vi "Get.vi"(8 "error in (no error)":errorcluster, 10 "uService ID":string, 11 "Distr uS Map ref in":refnum<data-value>) -> (0 "error out":errorcluster, 1 "uService found?":bool=TRUE, 2 "Guardians":string[](array[string]), 3 "Distr uS Map ref out":refnum<data-value>)   [LabVIEW 2026, in "TALOS.lvlib" / "Classes.lvlib" / "Distributed uService Map.lvclass"]
uses:
  Distributed uService Map.lvclass
  Distributed uService Map.lvclass/Distributed uService Map.ctl
  Ancestor/Ancestor/Ancestor.lvclass/Ancestor.ctl
  FGV/Error Memory/Get Error Description.vi
  Support VIs/Get PC name.vi
  Ancestor/Ancestor/Read ID.vi
  Support VIs/Get Class Name.vi
  <vilib>/Utility/error.llb/Clear Errors.vi
  FGV/Error Memory/Error Memory Core.vi
  <vilib>/AdvancedString/Delimited String to 1D String Array.vi
  <vilib>/AdvancedString/Delimited String to 1D String Array (string).vi
  Support VIs/Circus Root Path.vi
  FGV/Error Memory/Error Crt Lvl checker.vi
  FGV/Error Memory/Error Memory Core.vi/40c8088d-b597-4017-91af-faa98e00292e.vi
  FGV/Error Memory/Error Memory Core.vi/d4a3ab98-063c-4e44-b43d-fbdcfe6c2be2.vi
  Support VIs/Global Memory.vi
  <vilib>/Utility/LVClass/Get LV Class Name.vi
  Support VIs/Is in Packed Library.vi
  Support VIs/TALOS Root path.vi
  Support VIs/Read CSV worksheet.vi
  Support VIs/Global Constants.vi
  <vilib>/Utility/error.llb/General Error Handler.vi
  Support VIs/Error Log.vi
  Ancestor/Ancestor/Ancestor.lvclass
  <vilib>/Comparison/Equal/Equal Functor/Equal Functor.lvclass
  TALOS.lvlib
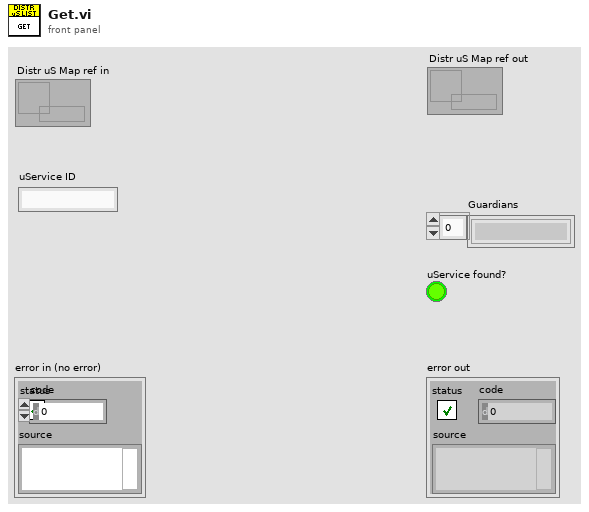
[diagram p1: front panel]
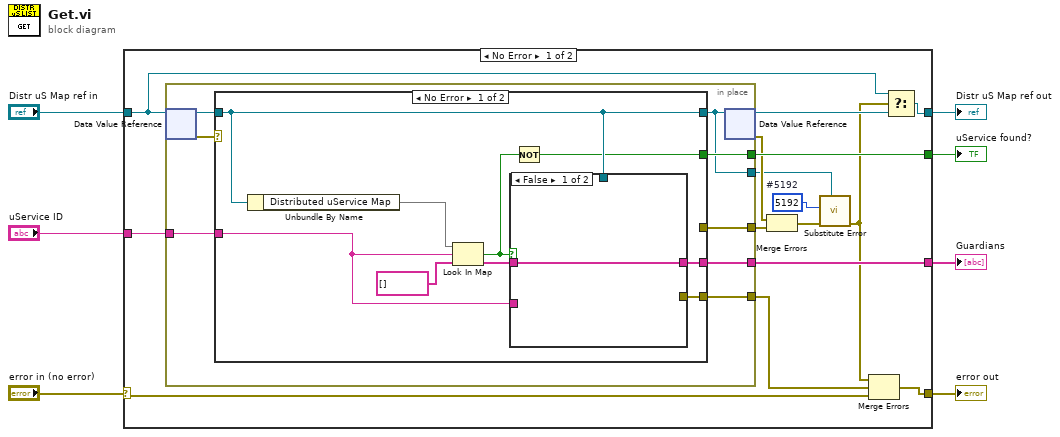
[diagram p0: block diagram]
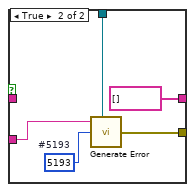
[diagram p2: hidden frame]
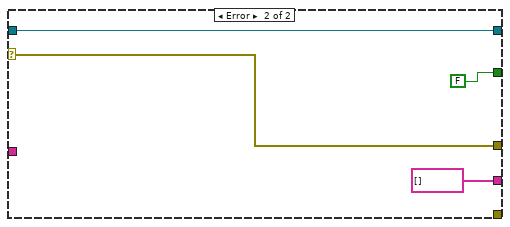
[diagram p3: hidden frame]
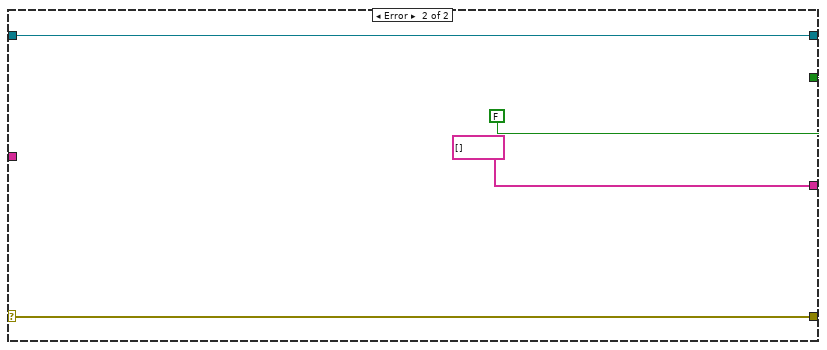
[diagram p4: hidden frame]
diagram:
  n1 = case shown="No Error" "error in (no error)" {
    selector: "error in (no error)" -> [w20 w53]
    tunnel: [w14 w53] -> w6
    tunnel: [w18 w52] -> w1
    tunnel: "Distr uS Map ref in" -> [w17 w52]
    tunnel: "uService ID" -> [w19 _]
    tunnel: [w22 string[] [] ("GD Owners")] -> w4
    tunnel: [w21 FALSE ("key not found?")] -> w3
    frame No Error {
      w11 = 5192  # #5192
      n2 = in-place {
        in-place-border: [w30] -> w22
        in-place-border: [w29] -> w21
        in-place-border: [w28] -> w15
        in-place-border: w19 -> [w27]
        in-place-border: [w24] -> w13
        in-place-border: [w23] -> w9
        n3 = in-place-dvr #1(w17) -> (w25:refnum<class "Distributed uService Map.lvclass">, w26:errorcluster)
        n4 = case shown="No Error" w26 {
          selector: w26 -> [_ w46]
          tunnel: [w36 string[] [] ("GD Owners")] -> w30
          tunnel: [w31 FALSE ("key not found?")] -> w29
          tunnel: [w34 _] -> w28
          tunnel: w27 -> [w33 _]
          tunnel: w25 -> [w32 w47]
          tunnel: [w32 w47] -> w23
          tunnel: [_ w46] -> w24
          frame No Error {
            n5 = Unbundle By Name(w32) -> ("Distributed uService Map"=w39:map{string, string[]})
            n6 = Look In Map(map=w39, key=w33, default value=string[] []) -> (key not found?=w35:bool, value=w37:string[])
            n7 = case shown="False" w35 {
              tunnel: [_ w44] -> w34
              tunnel: w37 -> [w40 _]
              tunnel: [w40 string[] []] -> w36
              tunnel: w33 -> [_ w42]
              tunnel: w32 -> [_ w41]
              frame False {
              }
              frame True {
                w45 = 5193  # #5193
                n8 = call "Generate Error.vi"("Optional String"=w42, "Class"=w41, "Error Code"=w45) -> ("error out"=w44:errorcluster)  [unwired: 4 in]
              }
            }
            n9 = Not(x=w35) -> (.not. x?=w31:bool)
          }
          frame Error {
          }
        }
        n10 = in-place-dvr #1(w23) -> (w16:refnum<data-value>, w12:errorcluster)
      }
      n11 = Merge Errors(w12, w13) -> (w10:errorcluster)
      n12 = call "Substitute Error.vi"("LabVIEW Object"=w9, "error in (no error)"=w10, "Error Code"=w11) -> ("error out"=w8:errorcluster)  [unwired: 8 in]
      n13 = Merge Errors(w8, w15, w20) -> (w14:errorcluster)
      n14 = Select(t=w17, s=w8, f=w16) -> (s? t:f=w18:refnum<data-value>)
    }
    frame Error {
    }
  }
  "error out" <- w6
  "Guardians" <- w4
  "uService found?" <- w3
  "Distr uS Map ref out" <- w1
